vi "Z6_Beamline.contents.vi"   [LabVIEW 2014, in "Z6_Beamline.lvlib"]
doc: "This class is forseen to inspect the PHELIX beamline and to select the mode. Additional several settings can be chosen.\n\nThis class is part of the PHELIX user layer."
uses:
  Z6_Beamline.lvlib
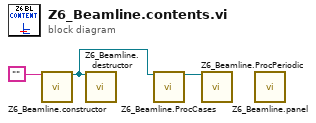
[diagram p0: block diagram]
diagram:
  n1 = call "Z6_Beamline.constructor.vi"("name"="") -> ("i ref out"=w1:refnum<vi>)  [unwired: 16 in, 2 out]
  n2 = call "Z6_Beamline.destructor.vi"("i ref in"=w1) -> ()  [unwired: 18 in, 1 out]
  n3 = call "Z6_Beamline.ProcCases.vi"("i ref in"=w1) -> ("i ref out"=w2:refnum<vi>)  [unwired: 16 in, 2 out]
  n4 = call "Z6_Beamline.ProcPeriodic.vi"("i ref in"=w2) -> ()  [unwired: 16 in, 3 out]
  n5 = call "Z6_Beamline.panel.vi"() -> ()  [unwired: 19 in, 1 out]
